vi "Init.vi"(8 "error in (no error)":errorcluster, 11 "Report In":refnum<class "Report Plugin.lvclass">) -> (0 "error out":errorcluster, 3 "Report Out":refnum<class "Report Plugin.lvclass">)   [LabVIEW 2020, in "Report Plugin.lvclass"]
uses:
  Report Plugin.lvclass
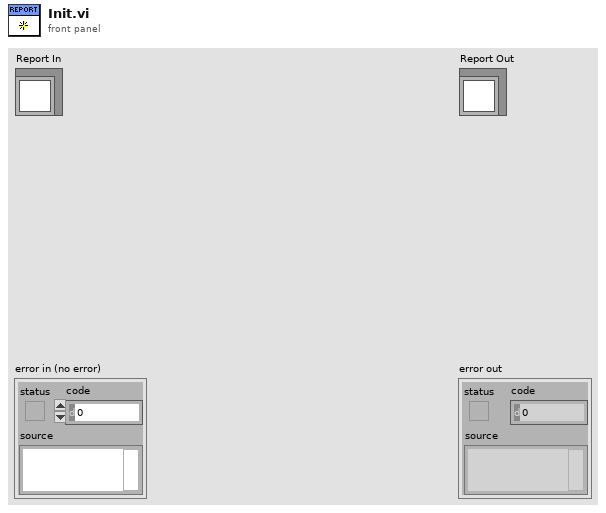
[diagram p1: front panel]
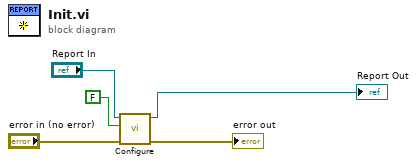
[diagram p0: block diagram]
diagram:
  n1 = call-dynamic "Configure.vi"("error in (no error)"="error in (no error)", "Interactive?"=FALSE, "Report Interface in"="Report In") -> ("error out"=→"error out":errorcluster, "Report Interface out"=→"Report Out":refnum<class "Report Plugin.lvclass">)  [unwired: 7 in]
